vi "G-Audio multi-device.vi"() -> ()   [LabVIEW 2020]
uses:
  <vilib>/Dataflow_G/G-Audio/Controls/Audio Device Config.ctl
  <vilib>/Dataflow_G/G-Audio/Controls/Audio Device Format.ctl
  c1cbce2a-475d-4e2a-9087-e8f963b6bf30.vi
  82cbf5ff-8e42-4bad-9895-649e6891c7ba.vi
  01849252-9acb-43f5-9470-b1ed8bc2d1dd.vi
  d8e41d60-1614-4341-92c7-01e77fb01fa2.vi
  a3ecb713-37bc-47d1-9ecb-ced5a3e47180.vi
  5da18835-cd31-4441-bb36-567579e18504.vi
  <vilib>/Dataflow_G/G-Audio/Private/Get Basic Audio File Info.vi
  <vilib>/Dataflow_G/G-Audio/Private/Result To Error.vi
  82cbf5ff-8e42-4bad-9895-649e6891c7ba.vi/4cbfd877-0a2d-4d89-9824-073e5c577ff5.vi
  <vilib>/Dataflow_G/G-Audio/Private/Audio File Refnum To Value.vi
  82cbf5ff-8e42-4bad-9895-649e6891c7ba.vi/909c8c34-e69f-4585-974e-b81a72aeefa8.vi
  <vilib>/Dataflow_G/G-Audio/Private/Audio Device Refnum To Value.vi
  01849252-9acb-43f5-9470-b1ed8bc2d1dd.vi/778ac659-2ffe-4b0a-adc6-ab59251bcc0d.vi
  01849252-9acb-43f5-9470-b1ed8bc2d1dd.vi/ca6afaa8-d499-43a3-87d2-894437d30b6f.vi
  a3ecb713-37bc-47d1-9ecb-ced5a3e47180.vi/4cbfd877-0a2d-4d89-9824-073e5c577ff5.vi
  a3ecb713-37bc-47d1-9ecb-ced5a3e47180.vi/909c8c34-e69f-4585-974e-b81a72aeefa8.vi
  5da18835-cd31-4441-bb36-567579e18504.vi/778ac659-2ffe-4b0a-adc6-ab59251bcc0d.vi
  5da18835-cd31-4441-bb36-567579e18504.vi/ca6afaa8-d499-43a3-87d2-894437d30b6f.vi
  82cbf5ff-8e42-4bad-9895-649e6891c7ba.vi/909c8c34-e69f-4585-974e-b81a72aeefa8.vi/47a590e7-b356-432c-9c8a-48a0405b5e18.vi
  01849252-9acb-43f5-9470-b1ed8bc2d1dd.vi/778ac659-2ffe-4b0a-adc6-ab59251bcc0d.vi/47a590e7-b356-432c-9c8a-48a0405b5e18.vi
  01849252-9acb-43f5-9470-b1ed8bc2d1dd.vi/ca6afaa8-d499-43a3-87d2-894437d30b6f.vi/67d3f12d-35d0-41d6-bcda-f56d91049287.vi
  a3ecb713-37bc-47d1-9ecb-ced5a3e47180.vi/909c8c34-e69f-4585-974e-b81a72aeefa8.vi/47a590e7-b356-432c-9c8a-48a0405b5e18.vi
  5da18835-cd31-4441-bb36-567579e18504.vi/778ac659-2ffe-4b0a-adc6-ab59251bcc0d.vi/47a590e7-b356-432c-9c8a-48a0405b5e18.vi
  5da18835-cd31-4441-bb36-567579e18504.vi/ca6afaa8-d499-43a3-87d2-894437d30b6f.vi/67d3f12d-35d0-41d6-bcda-f56d91049287.vi
  <vilib>/Dataflow_G/G-Audio/Audio Files/Polymorphic VIs/Get Audio File Info (Path).vi
  <vilib>/Dataflow_G/G-Audio/Audio Files/Polymorphic VIs/Open Audio File Read (Path).vi
  <vilib>/Utility/Data Type/Get Numeric Information.vi
  <vilib>/Utility/error.llb/Error Cluster From Error Code.vi
  <vilib>/Dataflow_G/G-Audio/G-Audio.lvlib
panel:
  in  "Device Selection":bool
  in  "Device 2":u16(ring) items=["Speakers (High Definition Audio Device)"]
  in  "Device":u16(ring) items=["Speakers (High Definition Audio Device)"]
  in  "Stop 2":bool
  out "Waveform 2":waveform(sgl)[](graph)
  out "error out 2":errorcluster
  out "Audio Info 2":T1
  out "Sample Length 2":u64
  out "Duration 2":string
  out "Now Playing: 2":string
  in  "Stop":bool
  out "Waveform":waveform(sgl)[](graph)
  out "error out":errorcluster
  out "Audio Info":T1
  out "Sample Length":u64
  out "Duration":string
  out "Now Playing:":string
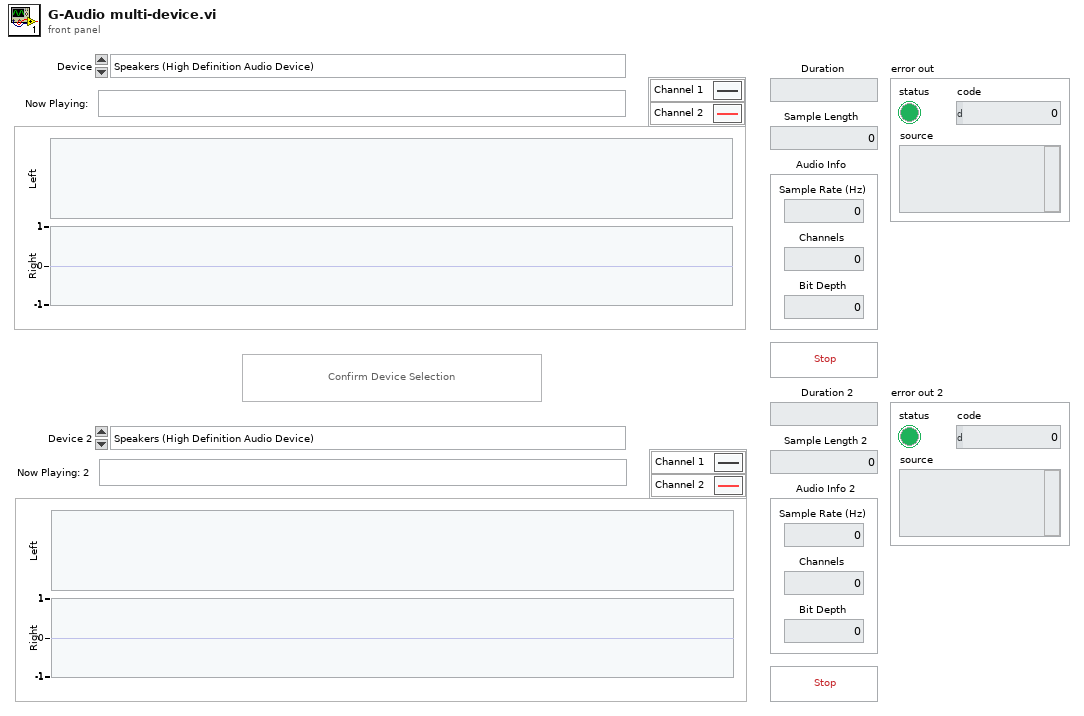
[diagram p1: front panel]
types:
  T1 = cluster{"Sample Rate (Hz)":u32, "Channels":u32, "Bit Depth":u32}
  T2 = enum8{"Enabled", "Disabled", "Disabled and Grayed Out"}
  T3 = typedef "G-Audio.lvlib/Audio Device Info.ctl" = cluster{"Name":string, "ID":u8[], "Device Type":T4}
  T4 = typedef "G-Audio.lvlib/Audio Device Type.ctl" = enum16{"(None)", "Playback", "Capture", "Duplex", "Loopback"}
  T5 = typedef "G-Audio.lvlib/Audio Device Config.ctl" = cluster{"Sample Rate (Hz)":u32, "Channels":u32, "Format":T6, "Exclusive Mode":bool}
  T6 = typedef "G-Audio.lvlib/Audio Device Format.ctl" = enum16{"Native", "U8", "I16", "I32", "SGL"}
  T7 = typedef "G-Audio.lvlib/Audio File Info.ctl" = cluster{"Sample Rate (Hz)":u32, "Channels":u32, "Bit Depth":u32}
  T8 = typedef "G-Audio.lvlib/Audio File Refnum.ctl" = refnum<file>
  T9 = typedef "G-Audio.lvlib/Audio Device Refnum.ctl" = refnum<file>
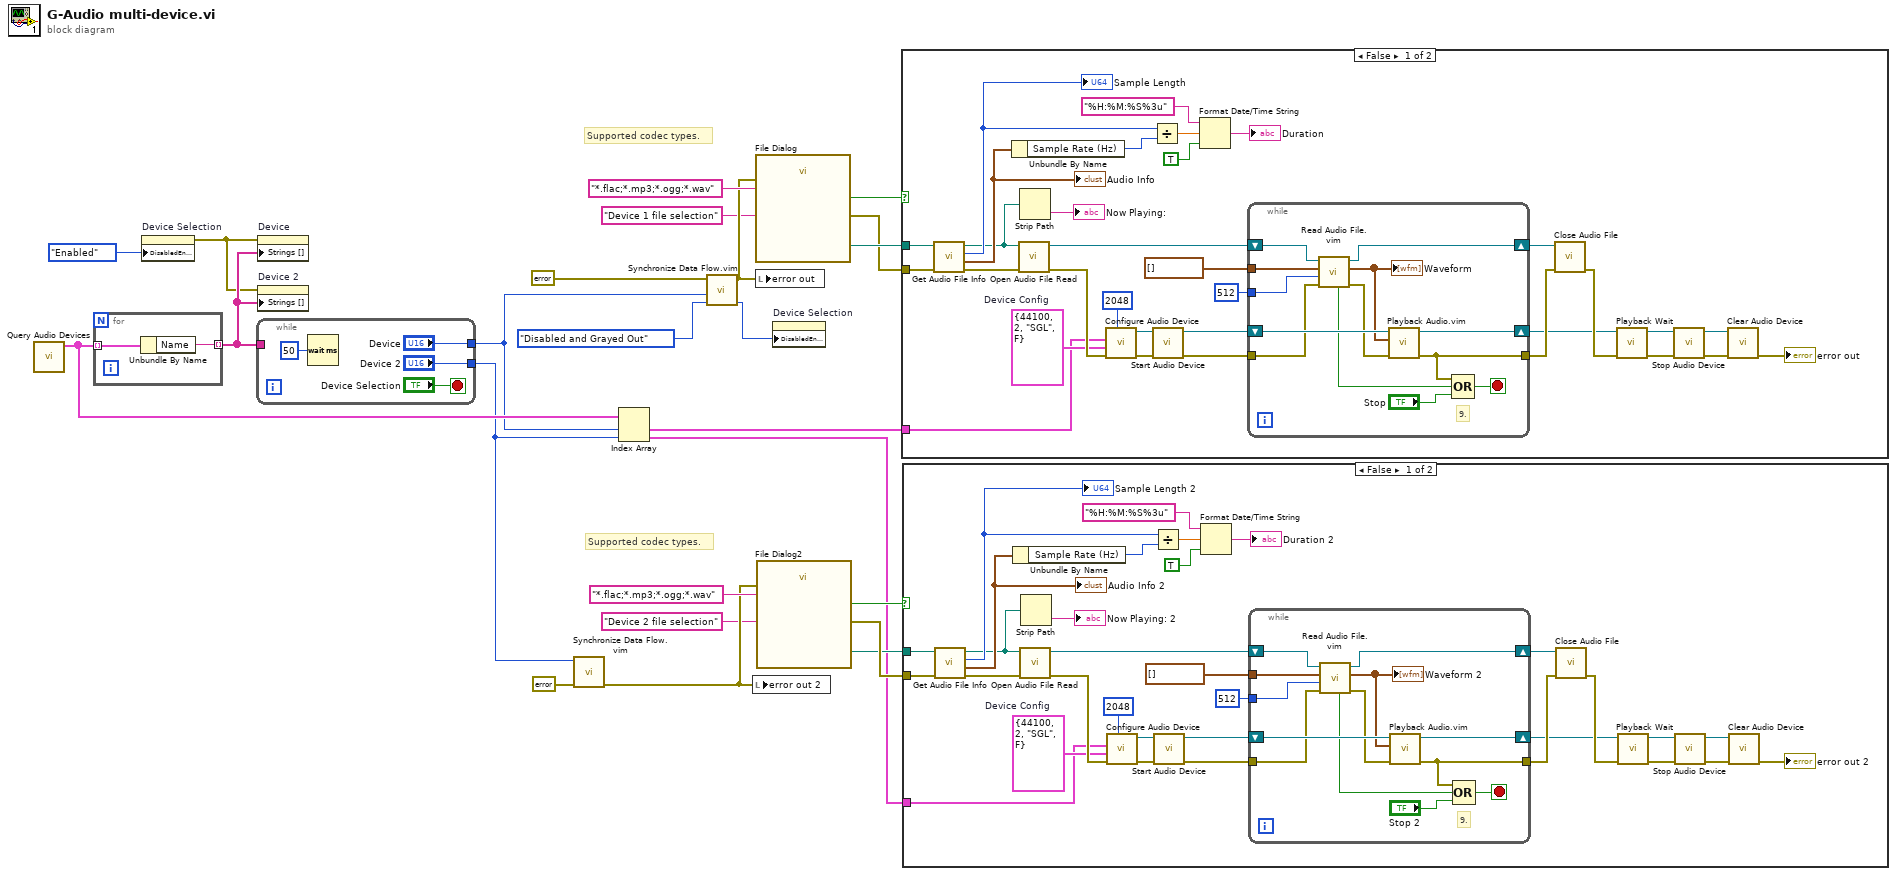
[diagram p0: block diagram]
diagram:
  # "Supported codec types."
  # "Supported codec types."
  n1 = call <vilib>:"Query Audio Devices.vi"() -> ("Playback Devices"=w15:T3[])  [unwired: 7 in, 4 out]
  n2 = for {
    tunnel: w15 -> [w26] mode=indexing
    tunnel: [w25] -> w16 mode=indexing
    n3 = Unbundle By Name(w26) -> ("Name"=w25:string)
  }
  n4 = property on="Device Selection" class="Bool"("DisabledEnum"=T2."Enabled" ("Disabled")) -> (error out=w1:errorcluster)  [unwired: 2 in, 1 out]
  n5 = while {
    tunnel: ["Device"] -> w6
    tunnel: ["Device 2"] -> w8
    tunnel: w16 -> [_]
    stop <- "Device Selection" stop-if-true
    n6 = Wait (ms)(milliseconds to wait=u32 50) -> ()  [unwired: 1 out]
  }
  n7 = property on="Device" class="Ring (strict)"(error in=w1, "Strings []"=w16) -> ()  [unwired: 1 in, 2 out]
  n8 = property on="Device 2" class="Ring (strict)"(error in=w1, "Strings []"=w16) -> ()  [unwired: 1 in, 2 out]
  n9 = call "Synchronize Data Flow.vim"("input 4"=errorcluster {"status"=FALSE, "code"=0, "source"=""} ("error out"), "input 1"=w8) -> ("output 4"=w9:errorcluster)  [unwired: 2 in, 3 out]
  n10 = Index Array(array=w15, index #1=w6, index #2=w8) -> (element #1=w14:T3, element #2=w13:T3)
  n11 = call "Synchronize Data Flow.vim"("input 4"=T2."Disabled and Grayed Out" ("Disabled"), "input 3"=w6, "input 1"=errorcluster {"status"=FALSE, "code"=0, "source"=""} ("error out")) -> ("output 4"=w4:T2, "output 1"=w11:errorcluster)  [unwired: 1 in, 2 out]
  n12 = local write "error out 2"(w9) -> ()
  n13 = call "File Dialog"("prompt"="Device 1 file selection", "error in"=w11, "pattern (all files)"="*.flac;*.mp3;*.ogg;*.wav") -> ("selected path"=w23:path, "cancelled"=w22:bool, "error out"=w21:errorcluster)  [unwired: 9 in, 1 out]
  n14 = local write "error out"(w11) -> ()
  n15 = call "File Dialog2"("prompt"="Device 2 file selection", "error in"=w9, "pattern (all files)"="*.flac;*.mp3;*.ogg;*.wav") -> ("selected path"=w18:path, "cancelled"=w19:bool, "error out"=w20:errorcluster)  [unwired: 9 in, 1 out]
  n16 = property on="Device Selection" class="Bool"("DisabledEnum"=w4) -> ()  [unwired: 2 in, 2 out]
  n17 = case shown="False" w22 {
    tunnel: w23 -> [w35 _]
    tunnel: w21 -> [w62 _]
    tunnel: w14 -> [w32 _]
    frame False {
      w38 = T5 {"Sample Rate (Hz)"=44100, "Channels"=2, "Format"=enum."SGL", "Exclusive Mode"=FALSE}  # Device Config
      n18 = call-poly <vilib>:"Get Audio File Info.vi"("error in (no error)"=w62, "Path In"=w35) -> ("error out"=w61:errorcluster, "Audio File Info"=w50:T7, "PCM Frame Length"=w51:u64, "Path Out"=w34:path)  [unwired: 5 in, 1 out]
      "Audio Info" <- w50
      "Sample Length" <- w51
      n19 = Unbundle By Name(w50) -> ("Sample Rate (Hz)"=w49:u32)
      n20 = call-poly <vilib>:"Open Audio File Read.vi"("error in (no error)"=w61, "Path"=w34) -> ("error out"=w39:errorcluster, "Audio File Refnum"=w53:T8)  [unwired: 8 in]
      n21 = Strip Path(path=w34) -> (name=→"Now Playing:":string)  [unwired: 1 out]
      n22 = call <vilib>:"Configure Audio Device.vi"("Buffer Size (4096)"=2048 ("number of samples/ch"), "error in (no error)"=w39, "Device Config"=w38, "Audio Device"=w32) -> ("error out"=w44:errorcluster, "Audio Device Refnum"=w43:T9)  [unwired: 6 in]
      n23 = Divide(x=w51, y=w49) -> (x/y=w48:dbl)
      n24 = call <vilib>:"Start Audio Device.vi"("error in (no error)"=w44, "Audio Device Refnum In"=w43) -> ("error out"=w54:errorcluster, "Audio Device Refnum Out"=w55:T9)  [unwired: 8 in]
      n25 = Format Date/Time String(time format string (%c)="%H:%M:%S%3u", seconds (now)=w48, UTC format=TRUE) -> (date/time string=→"Duration":string)
      n26 = while {
        shift-right: [w73] -> w60
        shift-left: w53 -> [w75]
        shift-right: [w72] -> w41
        shift-left: w55 -> [w74]
        tunnel: w54 -> [w71]
        tunnel: [w66] -> w58
        tunnel: u64 512 ("number of samples/ch") -> [w65]
        tunnel: waveform(sgl)[] [] -> [w64]
        stop <- w68 stop-if-true
        # "9."
        n27 = call "Read Audio File.vim"("error in (no error)"=w71, "Frames To Read"=w65, "Data Format"=w64, "Audio File Refnum In"=w75) -> ("error out"=w70:errorcluster, "Audio Data"=w63:waveform(sgl)[], "Audio File Refnum Out"=w73:T8, "End of File?"=w69:bool)  [unwired: 3 in, 1 out]
        "Waveform" <- w63
        n28 = call "Playback Audio.vim"("error in (no error)"=w70, "Audio Data"=w63, "Audio Device Refnum In"=w74) -> ("error out"=w66:errorcluster, "Audio Device Refnum Out"=w72:T9)  [unwired: 7 in]
        n29 = Compound Arithmetic op=OR(w66, w69, "Stop") -> (w68:bool)
      }
      n30 = call <vilib>:"Close Audio File.vi"("error in (no error)"=w58, "Audio File Refnum In"=w60) -> ("error out"=w57:errorcluster)  [unwired: 9 in]
      n31 = call <vilib>:"Playback Wait.vi"("error in (no error)"=w57, "Audio Device Refnum In"=w41) -> ("error out"=w42:errorcluster, "Audio Device Refnum Out"=w40:T9)  [unwired: 8 in]
      n32 = call <vilib>:"Stop Audio Device.vi"("error in (no error)"=w42, "Audio Device Refnum In"=w40) -> ("error out"=w56:errorcluster, "Audio Device Refnum Out"=w59:T9)  [unwired: 8 in]
      n33 = call <vilib>:"Clear Audio Device.vi"("error in (no error)"=w56, "Audio Device Refnum In"=w59) -> ("error out"=→"error out":errorcluster)  [unwired: 9 in]
    }
    frame True {
    }
  }
  n34 = case shown="False" w19 {
    tunnel: w18 -> [w80 _]
    tunnel: w20 -> [w107 _]
    tunnel: w13 -> [w77 _]
    frame False {
      w83 = T5 {"Sample Rate (Hz)"=44100, "Channels"=2, "Format"=enum."SGL", "Exclusive Mode"=FALSE}  # Device Config
      n35 = call-poly <vilib>:"Get Audio File Info.vi"("error in (no error)"=w107, "Path In"=w80) -> ("error out"=w106:errorcluster, "Audio File Info"=w95:T7, "PCM Frame Length"=w96:u64, "Path Out"=w79:path)  [unwired: 5 in, 1 out]
      "Audio Info 2" <- w95
      "Sample Length 2" <- w96
      n36 = Unbundle By Name(w95) -> ("Sample Rate (Hz)"=w94:u32)
      n37 = call-poly <vilib>:"Open Audio File Read.vi"("error in (no error)"=w106, "Path"=w79) -> ("error out"=w84:errorcluster, "Audio File Refnum"=w98:T8)  [unwired: 8 in]
      n38 = Strip Path(path=w79) -> (name=→"Now Playing: 2":string)  [unwired: 1 out]
      n39 = call <vilib>:"Configure Audio Device.vi"("Buffer Size (4096)"=2048 ("number of samples/ch"), "error in (no error)"=w84, "Device Config"=w83, "Audio Device"=w77) -> ("error out"=w89:errorcluster, "Audio Device Refnum"=w88:T9)  [unwired: 6 in]
      n40 = Divide(x=w96, y=w94) -> (x/y=w93:dbl)
      n41 = call <vilib>:"Start Audio Device.vi"("error in (no error)"=w89, "Audio Device Refnum In"=w88) -> ("error out"=w99:errorcluster, "Audio Device Refnum Out"=w100:T9)  [unwired: 8 in]
      n42 = Format Date/Time String(time format string (%c)="%H:%M:%S%3u", seconds (now)=w93, UTC format=TRUE) -> (date/time string=→"Duration 2":string)
      n43 = while {
        shift-right: [w118] -> w105
        shift-left: w98 -> [w120]
        shift-right: [w117] -> w86
        shift-left: w100 -> [w119]
        tunnel: w99 -> [w116]
        tunnel: [w111] -> w103
        tunnel: u64 512 ("number of samples/ch") -> [w110]
        tunnel: waveform(sgl)[] [] -> [w109]
        stop <- w113 stop-if-true
        # "9."
        n44 = call "Read Audio File.vim"("error in (no error)"=w116, "Frames To Read"=w110, "Data Format"=w109, "Audio File Refnum In"=w120) -> ("error out"=w115:errorcluster, "Audio Data"=w108:waveform(sgl)[], "Audio File Refnum Out"=w118:T8, "End of File?"=w114:bool)  [unwired: 3 in, 1 out]
        "Waveform 2" <- w108
        n45 = call "Playback Audio.vim"("error in (no error)"=w115, "Audio Data"=w108, "Audio Device Refnum In"=w119) -> ("error out"=w111:errorcluster, "Audio Device Refnum Out"=w117:T9)  [unwired: 7 in]
        n46 = Compound Arithmetic op=OR(w111, w114, "Stop 2") -> (w113:bool)
      }
      n47 = call <vilib>:"Close Audio File.vi"("error in (no error)"=w103, "Audio File Refnum In"=w105) -> ("error out"=w102:errorcluster)  [unwired: 9 in]
      n48 = call <vilib>:"Playback Wait.vi"("error in (no error)"=w102, "Audio Device Refnum In"=w86) -> ("error out"=w87:errorcluster, "Audio Device Refnum Out"=w85:T9)  [unwired: 8 in]
      n49 = call <vilib>:"Stop Audio Device.vi"("error in (no error)"=w87, "Audio Device Refnum In"=w85) -> ("error out"=w101:errorcluster, "Audio Device Refnum Out"=w104:T9)  [unwired: 8 in]
      n50 = call <vilib>:"Clear Audio Device.vi"("error in (no error)"=w101, "Audio Device Refnum In"=w104) -> ("error out"=→"error out 2":errorcluster)  [unwired: 9 in]
    }
    frame True {
    }
  }
